vi "Create BuildSpec Job.vi"(5 "Job.BuildSpec in":refnum<class "Job.BuildSpec.lvclass">, 6 "JobReport type":refnum<class "JobReport.lvclass">, 7 "Job Name":string, 8 "error in (no error)":errorcluster) -> (0 "error out":errorcluster, 3 "Job.BuildSpec":refnum<class "Job.BuildSpec.lvclass">)   [LabVIEW 2013, in "Job.BuildSpec.lvclass"]
uses:
  Job.BuildSpec.lvclass
  <vilib>/LabVIEW Open Source Project/Cron Scheduler/JobReport/JobReport.lvclass
  <vilib>/LabVIEW Open Source Project/Cron Scheduler/Job/Job.lvclass
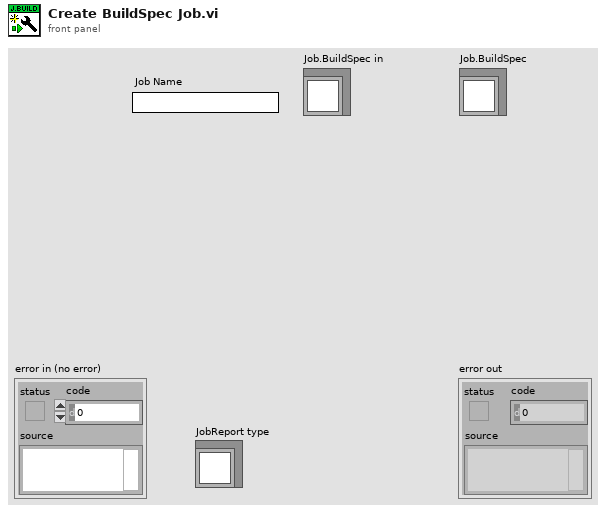
[diagram p1: front panel]
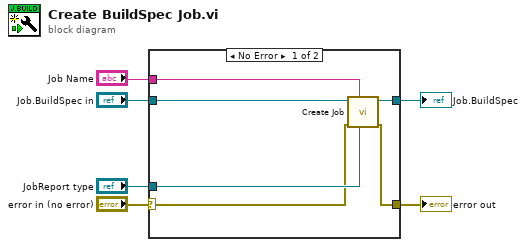
[diagram p0: block diagram]
diagram:
  n1 = case shown="No Error" "error in (no error)" {
    selector: "error in (no error)" -> [w9 w14]
    tunnel: [w8 w14] -> w5
    tunnel: [w12 w13] -> w3
    tunnel: "Job.BuildSpec in" -> [w7 w13]
    tunnel: "Job Name" -> [w11 _]
    tunnel: "JobReport type" -> [w10 _]
    frame No Error {
      n2 = call <vilib>:"Create Job.vi"("JobReport type"=w10, "Job Name"=w11, "error in (no error)"=w9, "Job in"=w7) -> ("error out"=w8:errorcluster, "Job"=w12:refnum<class "Job.BuildSpec.lvclass">)  [unwired: 6 in]
    }
    frame Error {
    }
  }
  "error out" <- w5
  "Job.BuildSpec" <- w3
